vi "Write ROI Name.vi"(8 "error in (no error)":errorcluster, 10 "ROI Name":string, 11 "Select Report File Dialog in":refnum<class "ROI Name Dialog.lvclass">) -> (0 "error out":errorcluster, 3 "Select Report File Dialog out":refnum<class "ROI Name Dialog.lvclass">)   [LabVIEW 2014, in "ROI Name Dialog.lvlib" / "ROI Name Dialog.lvclass"]
uses:
  ROI Name Dialog.lvclass
  ROI Name Dialog.lvclass/ROI Name Dialog.ctl
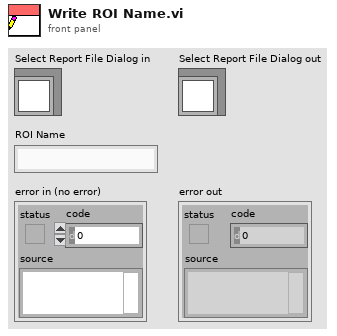
[diagram p1: front panel]
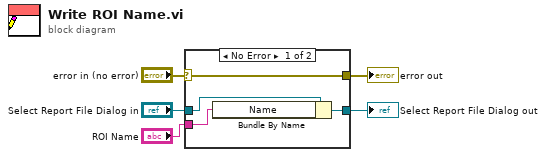
[diagram p0: block diagram]
diagram:
  n1 = case shown="No Error" "error in (no error)" {
    selector: "error in (no error)" -> [w9 w10]
    tunnel: [w9 w10] -> w4
    tunnel: [w7 w11] -> w2
    tunnel: "Select Report File Dialog in" -> [w8 w11]
    tunnel: "ROI Name" -> [w6 _]
    frame No Error {
      n2 = Bundle By Name(cluster=w8, "Name"=w6) -> (w7:refnum<class "ROI Name Dialog.lvclass">)
    }
    frame Error {
    }
  }
  "error out" <- w4
  "Select Report File Dialog out" <- w2
